vi "determineParametersFilePath.vi"(8 "error in (no error)":errorcluster, 11 "Logger in":refnum<class "Log.lvclass">) -> (0 "error out":errorcluster, 3 "Logger out":refnum<class "Log.lvclass">)   [LabVIEW 2013, in "Log.lvlib" / "Log.lvclass"]
uses:
  <userlib>/Common/Log/Log/Log.lvclass
  <userlib>/Common/Log/Log/Log.lvclass/Log.ctl
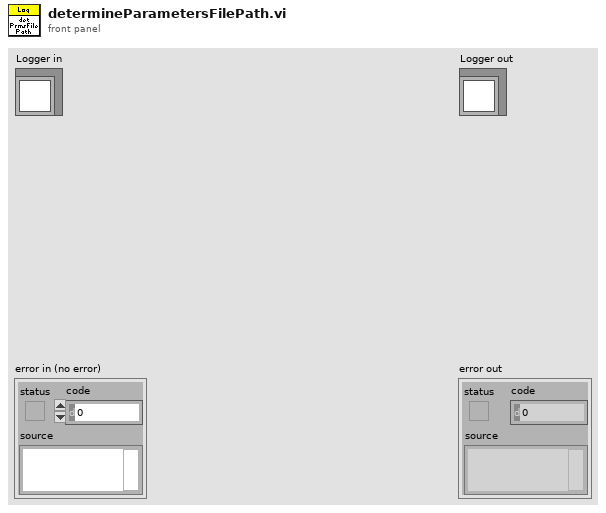
[diagram p1: front panel]
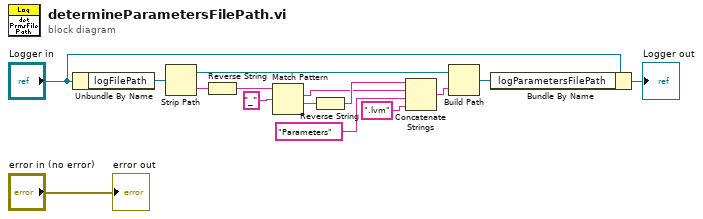
[diagram p0: block diagram]
diagram:
  n1 = Unbundle By Name("Logger in") -> ("logFilePath"=w2:path)
  n2 = Strip Path(path=w2) -> (stripped path=w8:path, name=w14:string)
  n3 = Reverse String(1:w14) -> (0:w13:string)
  n4 = Match Pattern(string=w13, regular expression="_") -> (match substring=w6:string, after substring=w7:string)  [unwired: 1 in, 2 out]
  n5 = Reverse String(1:w7) -> (0:w11:string)
  n6 = Concatenate Strings(w11, w6, "Parameters" ("string"), ".lvm" ("string")) -> (w9:string)
  n7 = Build Path(base path=w8, name or relative path=w9) -> (appended path=w4:path)
  n8 = Bundle By Name(cluster="Logger in", "logParametersFilePath"=w4) -> (→"Logger out":refnum<class "Log.lvclass">)
  "error out" <- "error in (no error)"
